vi "HEWH Read Standard Test.vi"(11 "Test Data Path":path) -> (3 "Array":T1[](array[typedef]) {"Time" format="%<%H:%M:%S>t"})   [LabVIEW 2016]
uses:
  Type Definitions/PRAT Test.ctl
  Utility/Save File/File Setup (Public)/Type Definition/Save File HEWH Heating Control Mode.ctl
  Draw Water Specific/Type Definitions/Terminate Draw Conditions.ctl
  Type Definitions/HEWH Start Conditions.ctl
  Draw Water Specific/Type Definitions/Check Special Condtions.ctl
  Draw Water Specific/Type Definitions/HEWH Special Condition Check.ctl
  Type Definitions/HEWH Draw Flag ENUM.ctl
  <vilib>/Utility/error.llb/whitespace.ctl
  <vilib>/Utility/file.llb/Read Delimited Spreadsheet (string).vi
  Utility/Save File/File Setup.lvlib
panel:
  out "all rows":string[][](array[string])
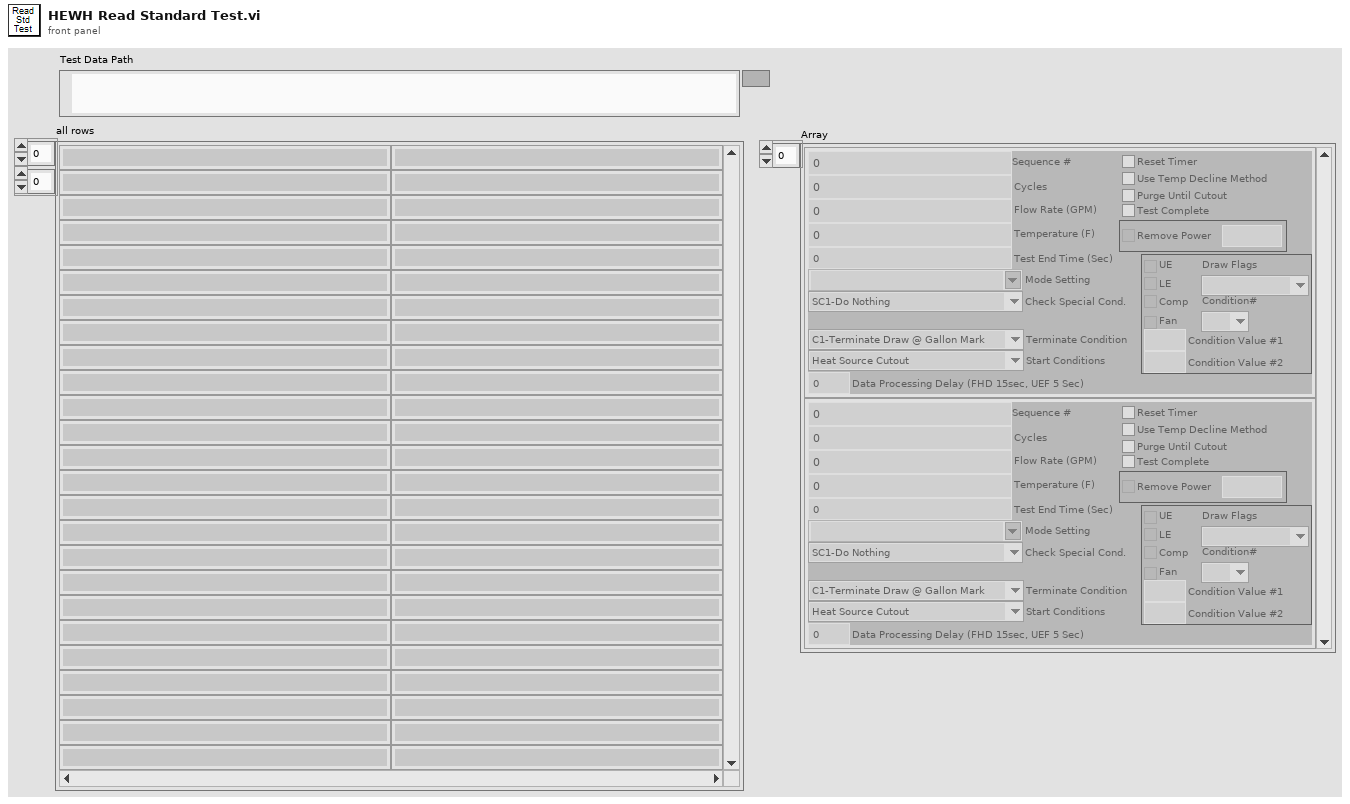
[diagram p1: front panel]
types:
  T1 = typedef "PRAT Test.ctl" = cluster{"Sequence #":dbl, "Cycles":i32, "Mode Setting":T2, "Flow Rate (GPM)":dbl, "Temperature (F)":dbl, "Reset Timer":bool, "Use Temp Decline Method":bool, "Terminate Condition":T3, "Condition Value #1":dbl, "UE":bool, "LE":bool, "Comp":bool, "Fan":bool, "Test End Time (Sec)":dbl, "Purge Until Cutout":bool, "Start Conditions":T4, "Condition Value #2":dbl, "Remove Power":bool, "Time":dbl, "Check Special Cond.":T5, "Condition#":T6, "Draw Flags":T7, "Data Processing Delay (FHD 15sec, UEF 5 Sec)":dbl, "Test Complete":bool}
  T2 = typedef "File Setup.lvlib/Save File HEWH Heating Control Mode.ctl" = string
  T3 = typedef "Terminate Draw Conditions.ctl" = enum16{"C1-Terminate Draw @ Gallon Mark", "C2-Special Last Draw (HU Test)", "C3-RTD Out <=", "C4-Mean Tank Temp <=", "C5-Decrease RTD Out (Deg F)", "C6-Time (Seconds)", "C7-Until Any Heat Source", "C8-Specific Heat Source", "C9-Do Nothing"}
  T4 = typedef "HEWH Start Conditions.ctl" = enum16{"Heat Source Cutout", "At Time (Seconds)", "Every X (Seconds)", "T2 >= X° Below Setpoint", "Seconds From Complete", "Wait for LE & Comp Cutout", "Wait for Comp Cutout", "Wait for LE Cutout", "Wait for UE Cutout"}
  T5 = typedef "Check Special Condtions.ctl" = enum16{"SC1-Do Nothing", "SC2-Check Heat Source (On-C2/Off-C1)", "SC3-Check Skip Condition", "SC4-Check Heat Source ON/Fail"}
  T6 = typedef "HEWH Special Condition Check.ctl" = enum16{"N/A", "C1", "C2", "Reset/Fail", "Skip Draw Sequence"}
  T7 = typedef "HEWH Draw Flag ENUM.ctl" = enum16{"N/A", "None(0)", "Sml(1)", "Med(2)", "SmlMed(3)", "Lrg(4)", "SmlLrg(5)", "MedLrg(6)", "SmlMedLrg(7)"}
  T8 = typedef "whitespace.ctl" = u16
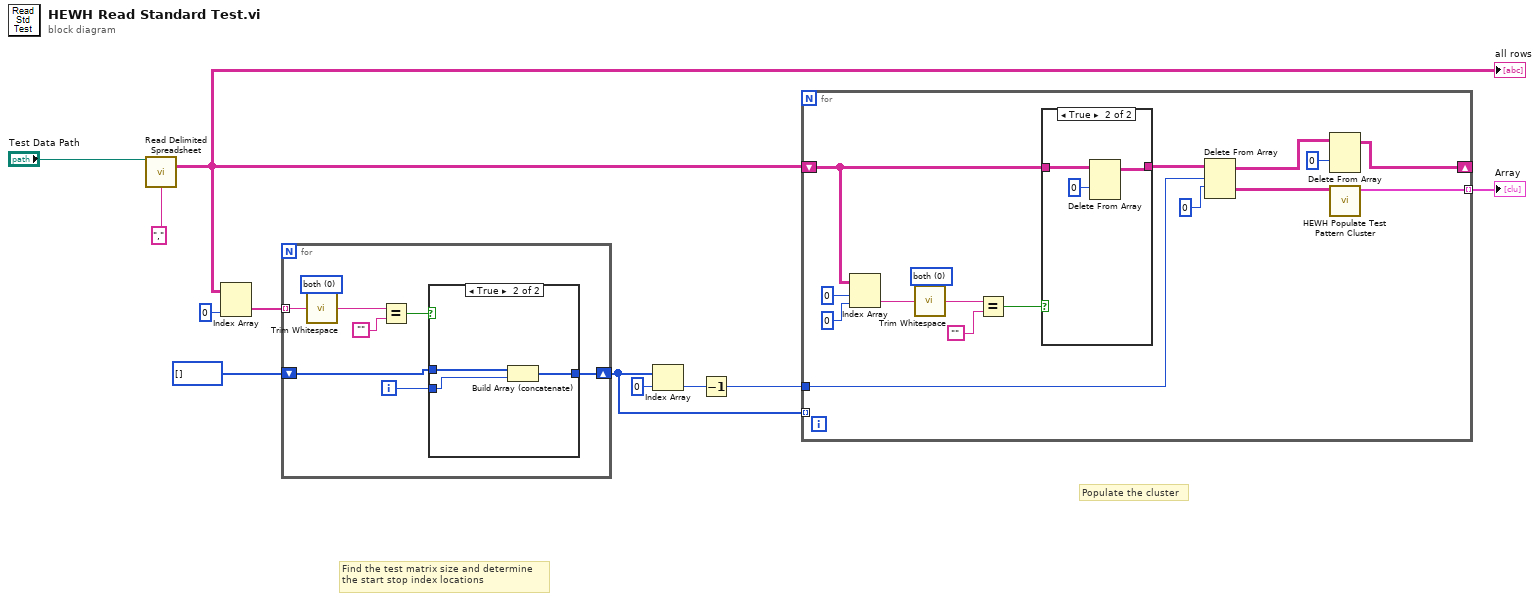
[diagram p0: block diagram]
diagram:
  # "Populate the cluster"
  # "Find the test matrix size and determine \nthe start stop index locations"
  n1 = call-poly <vilib>:"Read Delimited Spreadsheet.vi"("file path (dialog if empty)"="Test Data Path", "delimiter (\\t)"="," ("delimiter (\\t)")) -> ("all rows"=w9:string[][])  [unwired: 8 in, 5 out]
  "all rows" <- w9
  n2 = Index Array(array=w9, index (col)=0 ("disabled index (col)")) -> (element=w8:string[])  [unwired: 1 in]
  n3 = for {
    tunnel: w8 -> [w14] mode=indexing
    shift-right: [w16] -> w2
    shift-left: i32[] [] -> [w18]
    i -> [w15]
    w12 = T8 0 items=["both", "start of string", "end of string"] ("location (both)")
    n4 = call <vilib>:"Trim Whitespace.vi"("string"=w14, "location (both)"=w12) -> ("trimmed string"=w13:string)
    n5 = Equal?(x=w13, y="") -> (x = y?=w17:bool)
    n6 = case shown="True" w17 {
      tunnel: w18 -> [w20 w23]
      tunnel: [w20 w22] -> w16
      tunnel: w15 -> [_ w21]
      frame False {
      }
      frame True {
        n7 = Build Array (concatenate)(w23, w21) -> (w22:i32[])
      }
    }
  }
  n8 = Index Array(array=w2, index=0) -> (element=w4:i32)
  n9 = Decrement(x=w4) -> (x-1=w3:i32)
  n10 = for {
    tunnel: [w39] -> w1 mode=indexing
    tunnel: w3 -> [w38]
    shift-right: [w29] -> _
    shift-left: w9 -> [w28]
    tunnel: w2 -> [_] mode=indexing
    w26 = T8 0 items=["both", "start of string", "end of string"] ("location (both)")
    n11 = Index Array(array=w28, index (row)=0, index (col)=0 ("disabled index (col)")) -> (element=w27:string)
    n12 = call <vilib>:"Trim Whitespace.vi"("string"=w27, "location (both)"=w26) -> ("trimmed string"=w25:string)
    n13 = Equal?(x=w25, y="") -> (x = y?=w33:bool)
    n14 = case shown="True" w33 {
      tunnel: w28 -> [w40 w43]
      tunnel: [w40 w41] -> w32
      frame False {
      }
      frame True {
        n15 = Delete From Array(array=w43, index (row)=0) -> (array with subset deleted=w41:string[][])  [unwired: 2 in, 1 out]
      }
    }
    n16 = Delete From Array(array=w32, length=w38, index (row)=0 ("index")) -> (deleted portion=w24:string[][], array with subset deleted=w31:string[][])  [unwired: 1 in]
    n17 = Delete From Array(array=w31, index (row)=0) -> (array with subset deleted=w29:string[][])  [unwired: 2 in, 1 out]
    n18 = call "HEWH Populate Test Pattern Cluster.vi"("all rows"=w24) -> ("Cluster"=w39:T1)  [unwired: 9 in, 1 out]
  }
  "Array" <- w1
